vi "uService GUI.vi"(8 "error in (no error)":errorcluster, 11 "uService Template in":refnum<class "Pizza Machine.lvclass">) -> (3 "uService Template out":refnum<class "Pizza Machine.lvclass">)   [LabVIEW 2020, in "Pizza Machine.lvlib" / "Pizza Machine.lvclass"]
uses:
  Pizza Machine.lvclass
  C:/LabVIEW Code/aegis-labview-code/TALOS/TALOS_PPL.lvlibp/Father of all uServices/Father of all uServices/Father of all uServices.lvclass
  TALOS/TALOS_PPL.lvlibp/Father of all uServices/Father of all uServices/Father of all uServices.lvclass
  Pizza Machine.lvclass/Pizza Machine.ctl
panel:
  in  "Pizza flavour":string(combo)
  out "Order status":string
  in  "stop New uService":bool
  in  "Order Pizza":bool
  # "Pizza Machine"
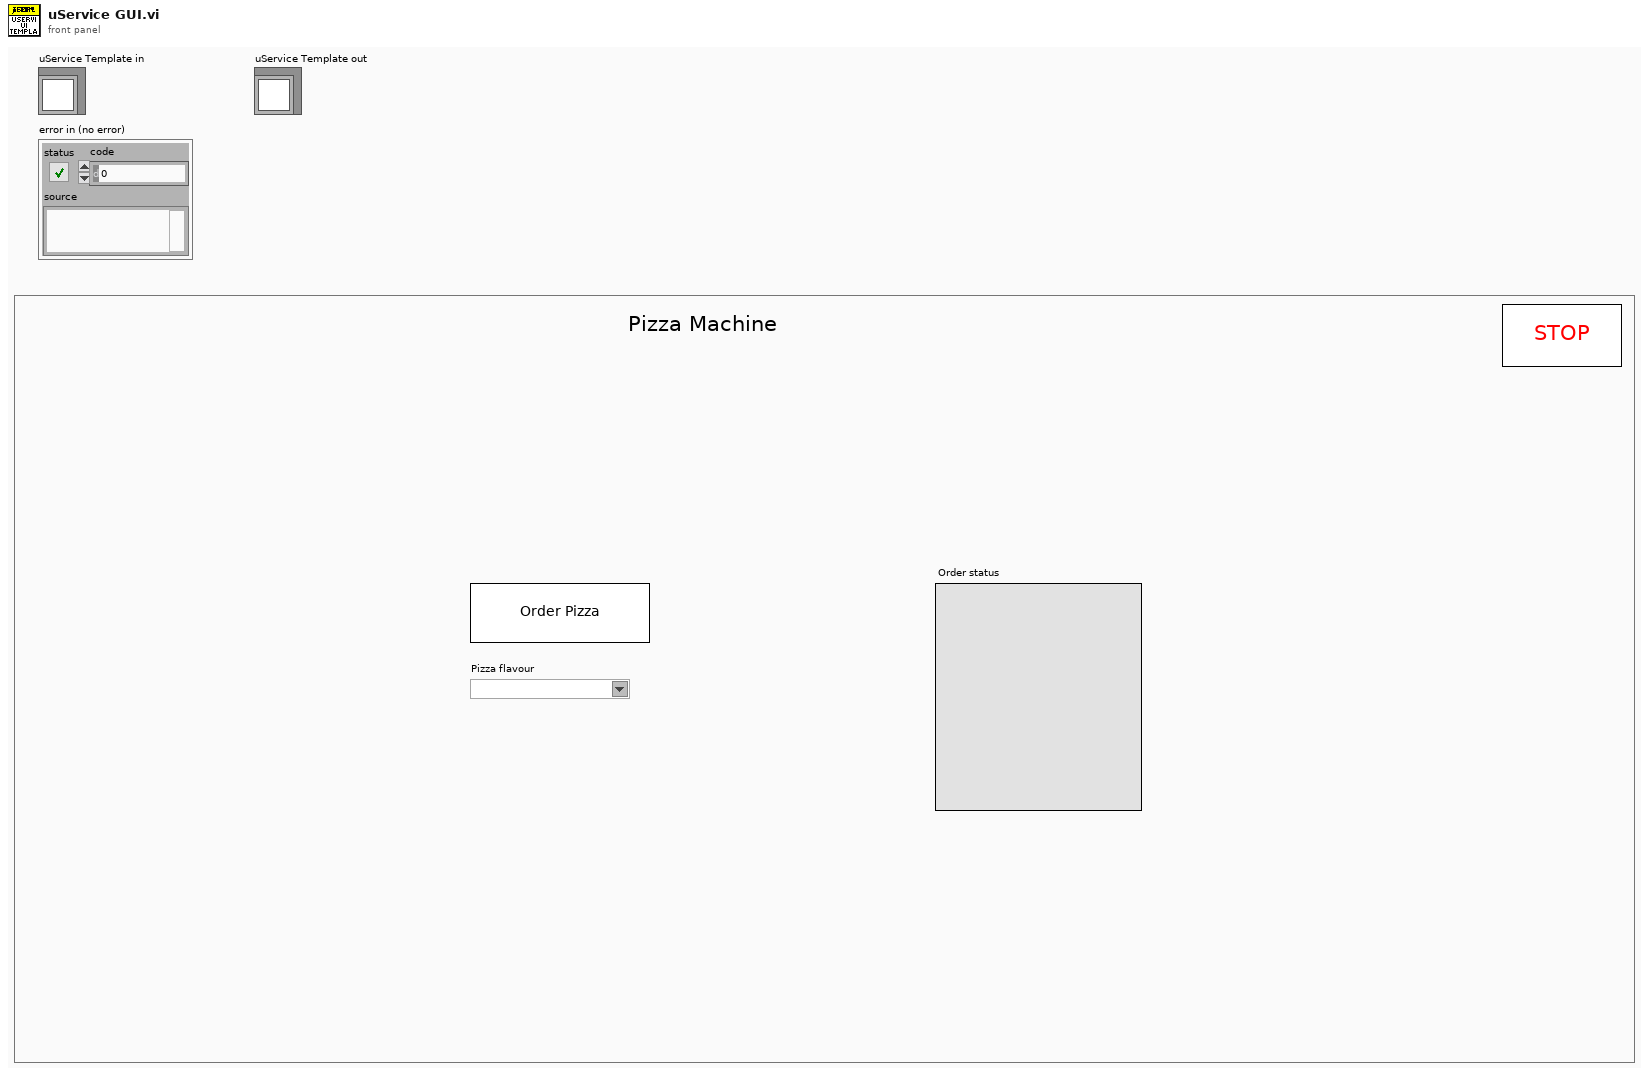
[diagram p1: front panel]
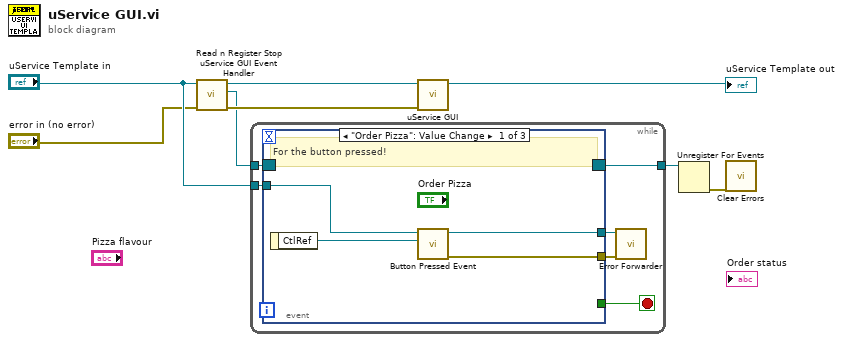
[diagram p0: block diagram]
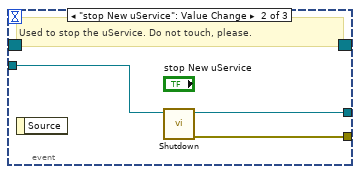
[diagram p2: hidden frame]
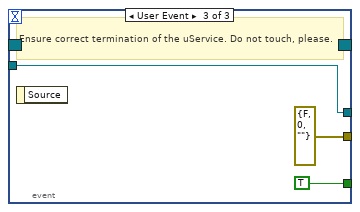
[diagram p3: hidden frame]
diagram:
  n1 = call-dynamic "Read n Register Stop uService GUI Event Handler .vi"("error in (no error)"="error in (no error)", "uService Template in"="uService Template in") -> ("error out"=w6:errorcluster, "Stop uService GUI Event Ref"=w5:refnum<event-registration>, "uService Template out"=w7:refnum<class "Pizza Machine.lvclass">)  [unwired: 7 in]
  n2 = while {
    tunnel: [w14] -> w8
    tunnel: w5 -> [w12]
    tunnel: "uService Template in" -> [w11]
    stop <- w13 stop-if-true
    n3 = event shown="[0] \"Order Pizza\": Value Change" {
      selector: w12 -> [_ _ _]
      dyn-events: [_ _ _] -> w14
      timeout: _ -> [_ _ _]
      tunnel: [_ _ TRUE] -> w13
      tunnel: w11 -> [w18 w21 w23]
      tunnel: [w16 w20 errorcluster {"status"=FALSE, "code"=0, "source"=""} ("error out")] -> w10
      tunnel: [w15 w19 w23] -> w9
      event "Order Pizza": Value Change {
        # "For the button pressed!"
        n4 = event-data() -> ("CtlRef"=w17:refnum<vi>)  [unwired: 1 in]
        n5 = call-dynamic "Button Pressed Event.vi"("CtlRef"=w17, "uService Template in"=w18) -> ("error out"=w16:errorcluster, "uService Template out"=w15:refnum<class "Pizza Machine.lvclass">)  [unwired: 8 in]
      }
      event "stop New uService": Value Change {
        # "Used to stop the uService. Do not touch, please."
        n6 = event-data() -> ()  [unwired: 1 in, 1 out]
        n7 = call "Shutdown.vi"("Father of all uServices in"=w21) -> ("error out"=w20:errorcluster, "Father of all uServices out"=w19:refnum<class "Pizza Machine.lvclass">)  [unwired: 9 in]
      }
      event User Event {
        # "Ensure correct termination of the uService. Do not touch, please."
        n8 = event-data() -> ()  [unwired: 1 in, 1 out]
      }
    }
    n9 = call "Error Forwarder.vi"("error in (no error)"=w10, "Father of all uServices in"=w9) -> ()  [unwired: 10 in]
  }
  n10 = call-parent "uService GUI.vi"("error in (no error)"=w6, "uService Template in"=w7) -> ("uService Template out"=→"uService Template out":refnum<class "Pizza Machine.lvclass">)  [unwired: 9 in]
  n11 = Unregister For Events(event registration refnum=w8) -> (error out=w1:errorcluster)  [unwired: 1 in]
  n12 = call <vilib>:"Clear Errors.vi"("error in (no error)"=w1) -> ()  [unwired: 5 in, 2 out]
